vi "Test_WriteItem_DeleteItemNoTypeCheck_ItemRemoved.vi"(8 "error in (no error)":errorcluster, 11 "TestCase in":refnum<class "TestComposedLookupTable.lvclass">) -> (0 "error out":errorcluster, 3 "TestCase out":refnum<class "TestComposedLookupTable.lvclass">)   [LabVIEW 2017, in "TestComposedLookupTable.lvclass"]
uses:
  TestComposedLookupTable.lvclass
  Source/LookupTable/LookupTable.lvclass/LookupTable.ctl
  125561d6-b269-49e5-b398-38c54022091b.vi
  588ba77a-721b-4cbd-ab0d-abf1703ce9df.vi
  6ea268bf-f804-414d-a6d8-9bb4563e246d.vi
  Source/LookupTable/Read Table Reference.vi
  125561d6-b269-49e5-b398-38c54022091b.vi/f85152ab-feab-4561-abdd-bf91576b5904.vi
  6ea268bf-f804-414d-a6d8-9bb4563e246d.vi/d1f20482-5f11-4bb5-8bba-25276c52ad7c.vi
  Source/LookupTable/LookupTable.lvclass
panel:
  out "Value":i32
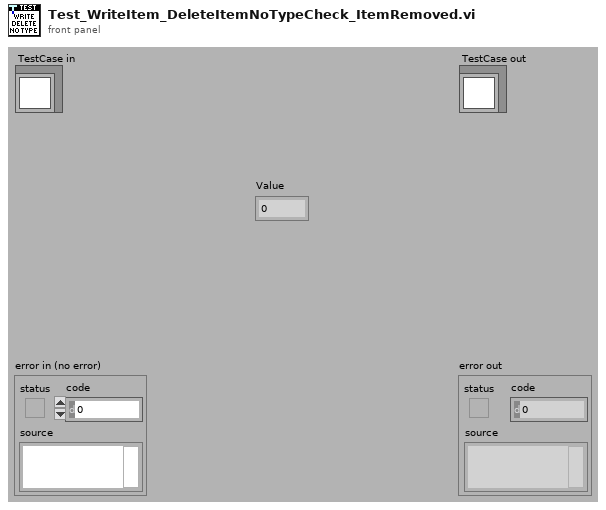
[diagram p1: front panel]
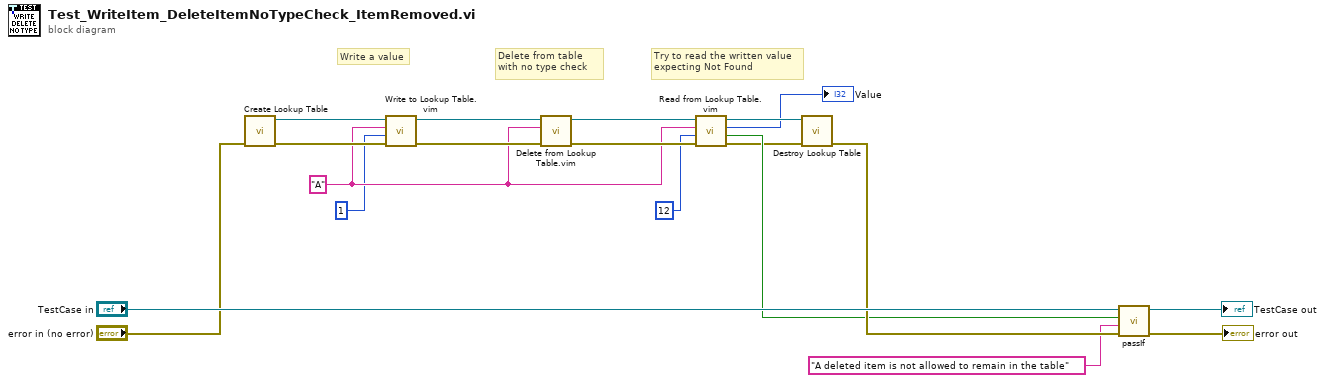
[diagram p0: block diagram]
diagram:
  w5 = "A" ("Item Name")
  # "Delete from table\nwith no type check"
  # "Try to read the written value\nexpecting Not Found"
  # "Write a value"
  n1 = call "Create Lookup Table.vi"("error in (no error)"="error in (no error)") -> ("error out"=w13:errorcluster, "LookupTable Reference"=w11:refnum<data-value>)  [unwired: 9 in]
  n2 = call "Write to Lookup Table.vim"("error in (no error)"=w13, "Item"=1, "Item Name"=w5, "LookupTable Reference"=w11) -> ("error out"=w12:errorcluster, "LookupTable Reference Out"=w7:refnum<data-value>)  [unwired: 5 in, 1 out]
  n3 = call "Delete from Lookup Table.vim"("error in (no error)"=w12, "Item Name"=w5, "LookupTable Reference"=w7) -> ("error out"=w8:errorcluster, "LookupTable Reference Out"=w6:refnum<data-value>)  [unwired: 6 in, 1 out]
  n4 = call "Read from Lookup Table.vim"("error in (no error)"=w8, "Type"=12, "Item Name"=w5, "LookupTable Reference"=w6) -> ("error out"=w9:errorcluster, "Not Found?"=w14:bool, "Value"=→"Value":i32, "LookupTable Reference Out"=w10:refnum<data-value>)  [unwired: 4 in]
  n5 = call "Destroy Lookup Table.vi"("error in (no error)"=w9, "LookupTable Reference"=w10) -> ("error out"=w15:errorcluster)  [unwired: 9 in]
  n6 = call-dynamic "passIf.vi"("error in (no error)"=w15, "message (\"\")"="A deleted item is not allowed to remain in the table" ("message (\"\")"), "pass"=w14, "TestCase in"="TestCase in") -> ("error out"=→"error out":errorcluster, "TestCase out"=→"TestCase out":refnum<class "TestComposedLookupTable.lvclass">)  [unwired: 6 in]
